vi "Read Channel Array.vi"(8 "error in":errorcluster, 10 "channels":refnum<class "Channel.lvclass">[](array[class]), 11 "digital input mode in":refnum<class "Digital Input and Output Mode.lvclass">) -> (0 "error out":errorcluster, 2 "channel settings":T1[](array[typedef]), 3 "digital input mode out":refnum<class "Digital Input and Output Mode.lvclass">)   [LabVIEW 2017]
uses:
  Digital Input and Output Mode.lvclass
  C:/dev/niveristand-scan-engine-ethercat-custom-device/Custom Device Source/Scripting/Modules/Mode Classes/Digital Mode/Digital Mode.lvclass
  Channel Classes/Channel/Channel.lvclass
  Controls/digital channel settings.ctl
  Digital Mode/Digital Mode.lvclass
  Scan Engine Scripting.lvlib
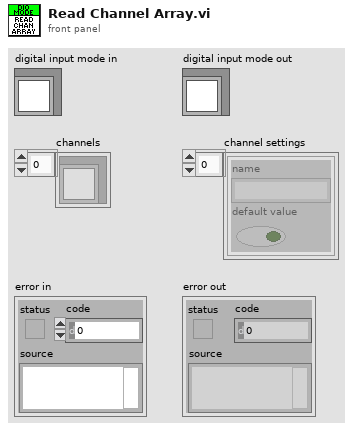
[diagram p1: front panel]
types:
  T1 = typedef "Scan Engine Scripting.lvlib/digital channel settings.ctl" = cluster{"name":string, "default value":bool}
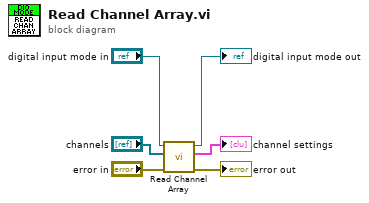
[diagram p0: block diagram]
diagram:
  n1 = call "Read Channel Array.vi"("error in"="error in", "channels"="channels", "digital mode in"="digital input mode in") -> ("error out"=→"error out":errorcluster, "channel settings"=→"channel settings":T1[], "digital mode out"=→"digital input mode out":refnum<class "Digital Input and Output Mode.lvclass">)  [unwired: 6 in]
